vi "check type and blank string.vi"(7 "default":string, 11 "user input":string) -> (3 "validated":string)   [LabVIEW 2013, in "data interface script.lvlib"]
uses:
  data interface script.lvlib
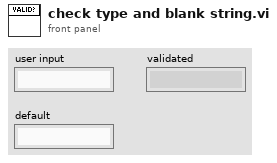
[diagram p1: front panel]
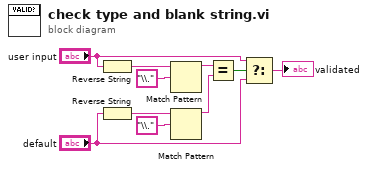
[diagram p0: block diagram]
diagram:
  n1 = Reverse String(1:"user input") -> (0:w7:string)
  n2 = Reverse String(1:"default") -> (0:w10:string)
  n3 = Match Pattern(string=w7, regular expression="\\.") -> (before substring=w6:string)  [unwired: 1 in, 3 out]
  n4 = Match Pattern(string=w10, regular expression="\\.") -> (before substring=w5:string)  [unwired: 1 in, 3 out]
  n5 = Equal?(x=w6, y=w5) -> (x = y?=w4:bool)
  n6 = Select(t="user input", s=w4, f="default") -> (s? t:f=→"validated":string)
